vi "Helper-ConvertRelativeWaypointToReal.vi"(9 "Current boat location":T1 {"North" format="%#_10f"; "East" format="%#_8f"}, 10 "Relative Waypoints In":cluster{"X":dbl, "Y":dbl}[](array[cluster])) -> (1 "Actual Waypoints Out":refnum<class "Waypoint.lvclass">[](array[class]))   [LabVIEW 2013]
uses:
  Data/TypeDefs/UTM Location.ctl
  Classes/Waypoint/Waypoint.lvclass
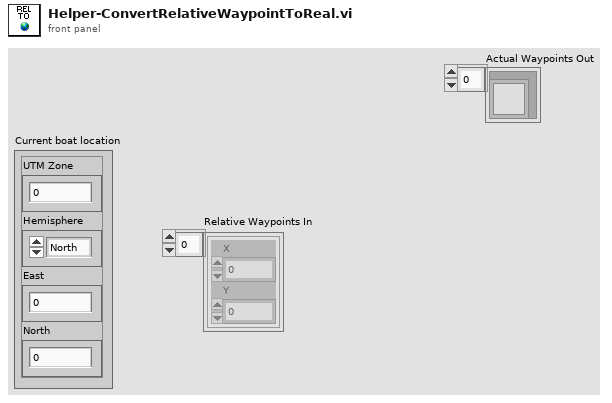
[diagram p1: front panel]
types:
  T1 = typedef "UTM Location.ctl" = cluster{"UTM Zone":dbl, "Hemisphere":enum16{"North", "South"}, "East":dbl, "North":dbl}
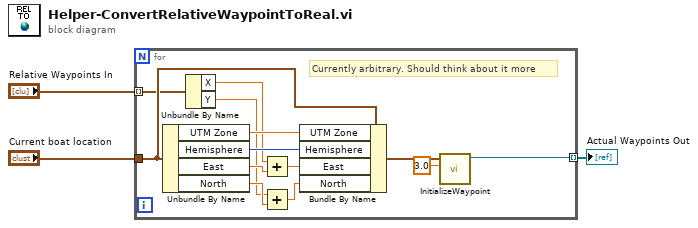
[diagram p0: block diagram]
diagram:
  n1 = for {
    tunnel: "Current boat location" -> [w14]
    tunnel: "Relative Waypoints In" -> [w9] mode=indexing
    tunnel: [w4] -> w1 mode=indexing
    # "Currently arbitrary. Should think about it more"
    n2 = Unbundle By Name(w14) -> ("UTM Zone"=w11:dbl, "Hemisphere"=w10:enum16{"North", "South"}, "East"=w16:dbl, "North"=w15:dbl)
    n3 = Unbundle By Name(w9) -> ("X"=w8:dbl, "Y"=w7:dbl)
    n4 = Add(x=w8, y=w16) -> (x+y=w13:dbl)
    n5 = Add(x=w7, y=w15) -> (x+y=w12:dbl)
    n6 = Bundle By Name(cluster=w14, "UTM Zone"=w11, "Hemisphere"=w10, "East"=w13, "North"=w12) -> (w6:T1)
    n7 = call "InitializeWaypoint.vi"("Tolerance (meters?) (0)"=3.0, "Coords"=w6) -> ("Waypoint Out"=w4:refnum<class "Waypoint.lvclass">)  [unwired: 9 in]
  }
  "Actual Waypoints Out" <- w1
